vi "CRYAPI TAB Get Tab Reference.vi"(8 "Label Name":string, 11 "VI Refnum":refnum<vi>) -> (1 "Boolean":bool, 2 "Tab Control Ref":refnum<vi>, 3 "VI Refnum Out":refnum<vi>)   [LabVIEW 2013]
panel:
  out "ActiveSubVI Number":i32
  out "VIRef_Draw 2":refnum<vi>[](array[refnum])
  out "SubVI Numeric":i32
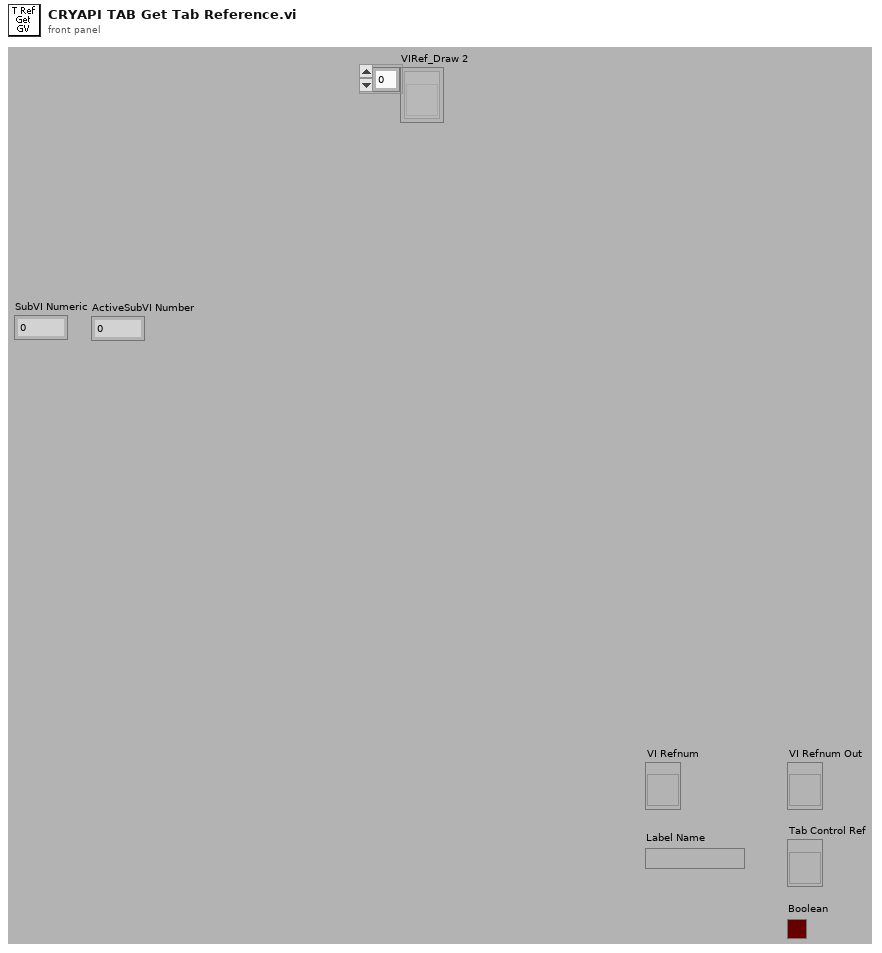
[diagram p1: front panel]
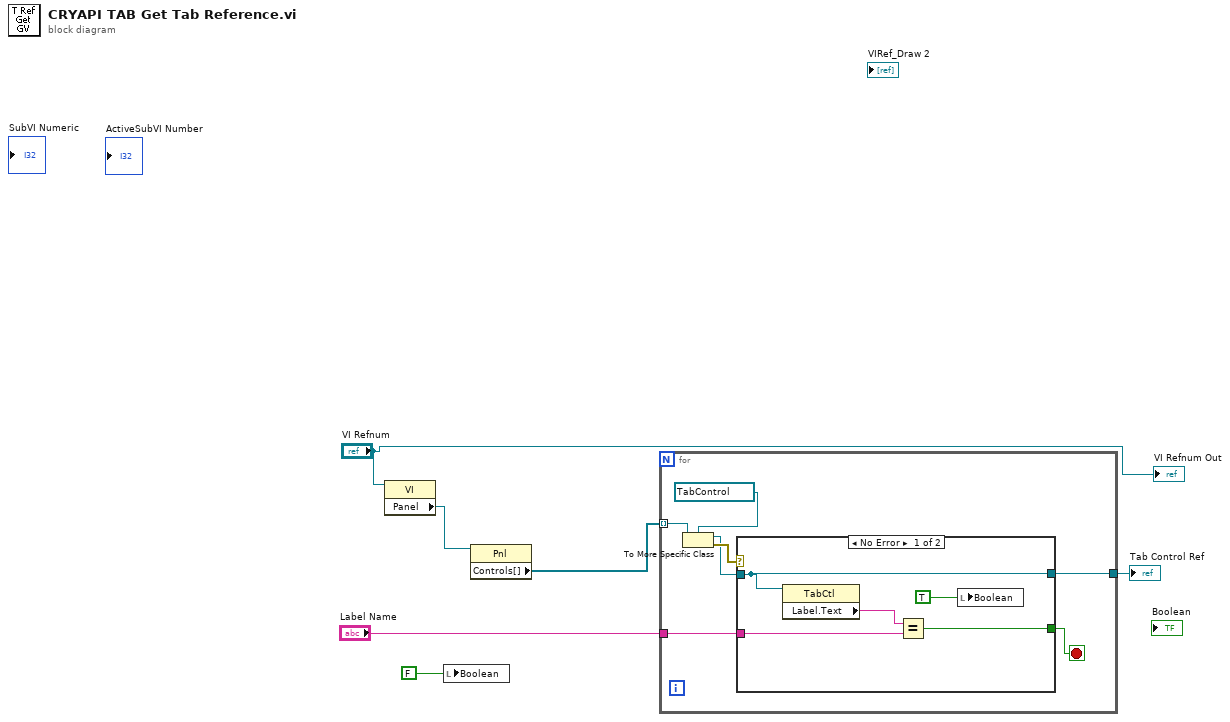
[diagram p0: block diagram]
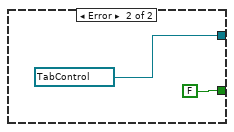
[diagram p2: hidden frame]
diagram:
  n1 = property class="VI"(reference="VI Refnum") -> ("Panel"=w4:refnum<vi>)  [unwired: 1 in, 2 out]
  n2 = local write "Boolean"(FALSE ("Boolean")) -> ()
  n3 = property class="Pnl"(reference=w4) -> ("Controls[]"=w3:refnum<vi>[])  [unwired: 1 in, 2 out]
  n4 = for {
    tunnel: w3 -> [w13] mode=indexing
    tunnel: [w9] -> w1
    tunnel: "Label Name" -> [w8]
    stop <- w10 stop-if-true
    n5 = To More Specific Class(target class=refnum<vi> refnum ("Tab Control"), reference=w13) -> (specific class reference=w11:refnum<vi>, error out=w12:errorcluster)  [unwired: 1 in]
    n6 = case shown="No Error" w12 {
      tunnel: w11 -> [w14 _]
      tunnel: [w17 FALSE] -> w10
      tunnel: [w14 refnum<vi> refnum ("Tab Control")] -> w9
      tunnel: w8 -> [w15 _]
      frame No Error {
        n7 = property class="TabCtl"(reference=w14) -> ("Label.Text"=w18:string)  [unwired: 1 in, 2 out]
        n8 = Equal?(x=w18, y=w15) -> (x = y?=w17:bool)
        n9 = local write "Boolean"(TRUE ("Boolean")) -> ()
      }
      frame Error {
      }
    }
  }
  "Tab Control Ref" <- w1
  "VI Refnum Out" <- "VI Refnum"
